vi "linearAccumulator.vi"(7 "reset":bool, 11 "input":i16) -> (3 "sum":i32)   [LabVIEW 2016]
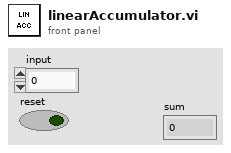
[diagram p1: front panel]
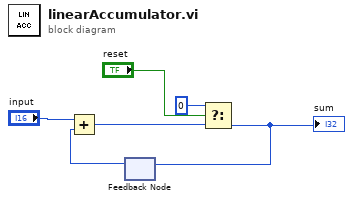
[diagram p0: block diagram]
diagram:
  n1 = feedback #1() -> (w6:i32)  [unwired: 1 in]
  n2 = Add(x="input", y=w6) -> (x+y=w5:i32)
  n3 = Select(t=0, s="reset", f=w5) -> (s? t:f=w3:i32)
  "sum" <- w3
  n4 = feedback-in #1(w3) -> ()
